vi "create.vi"(8 "error in":errorcluster, 10 "delay (s)":dbl) -> (0 "error out":errorcluster, 3 "comic_crawler.lvclass":refnum<class "comic_crawler.lvclass">)   [LabVIEW 2024, in "comic_crawler.lvclass"]
uses:
  comic_crawler.lvclass
  private/queue.message--cluster.ctl
  private/daemon.states--enum.ctl
  status--cluster.ctl
  comic_crawler.lvclass/comic_crawler.ctl
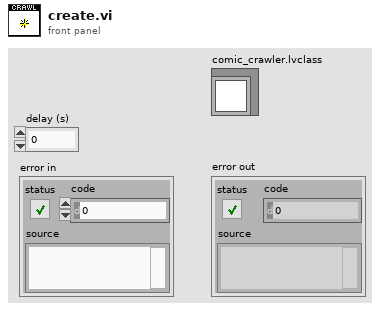
[diagram p1: front panel]
types:
  T1 = typedef "comic_crawler.lvclass/daemon.states--enum.ctl" = enum16{"start search", "idle", "set timer", "running", "stop search", "wait", "set delay", "shut down"}
  T2 = typedef "comic_crawler.lvclass/status--cluster.ctl" = cluster{"total files":i32, "comleted files":i32, "current file":string, "current state":string, "iteration":i32, "error status":errorcluster, "file queue size":i32, "Approx Completion":timestamp}
  T3 = typedef "comic_crawler.lvclass/queue.message--cluster.ctl" = cluster{"cmd":T1, "data":variant}
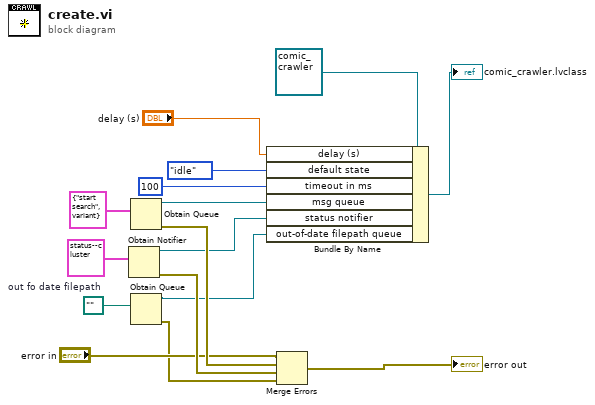
[diagram p0: block diagram]
diagram:
  w5 = path ""  # out fo date filepath
  n1 = Obtain Notifier(notification data type=T2 {"total files"=0, "comleted files"=0, "current file"="", "current state"="", "iteration"=0, "error status"={"status"=FALSE, "code"=0, "source"=""}, "file queue size"=0, "Approx Completion"=timestamp(0 s since 1904-01-01)} ("status")) -> (notifier out=w8:refnum<notifier>, error out=w7:errorcluster)  [unwired: 3 in, 1 out]
  n2 = Obtain Queue(element data type=T3 {"cmd"=enum."start search", "data"=variant} ("message")) -> (queue out=w14:refnum<queue>, error out=w11:errorcluster)  [unwired: 4 in, 1 out]
  n3 = Obtain Queue(element data type=w5) -> (queue out=w4:refnum<queue>, error out=w3:errorcluster)  [unwired: 4 in, 1 out]
  n4 = Bundle By Name(cluster=refnum<class "comic_crawler.lvclass"> refnum ("comic_crawler.lvclass"), "delay (s)"="delay (s)", "default state"=daemon.states--enum."idle" ("cmd"), "timeout in ms"=100, "msg queue"=w14, "status notifier"=w8, "out-of-date filepath queue"=w4) -> (→"comic_crawler.lvclass":refnum<class "comic_crawler.lvclass">)
  n5 = Merge Errors("error in", w11, w7, w3) -> (→"error out":errorcluster)
